vi "HTTP-Read Response.vi"(8 "error in (no error)":errorcluster, 11 "TCP Network Connection in":refnum<k5>) -> (0 "error out":errorcluster, 1 "Body":string, 2 "Header":string, 3 "TCP Network Connection out":refnum<k5>)   [LabVIEW 2020]
uses:
  <vilib>/regexp/Match Regular Expression.xnode
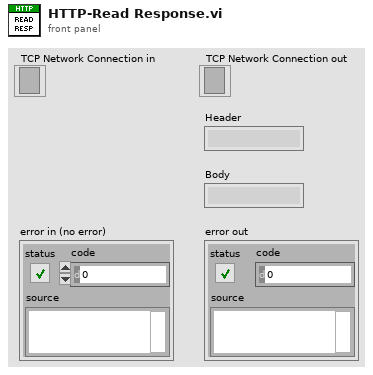
[diagram p1: front panel]
types:
  T1 = enum16{"Standard", "Buffered", "CRLF", "Immediate"}
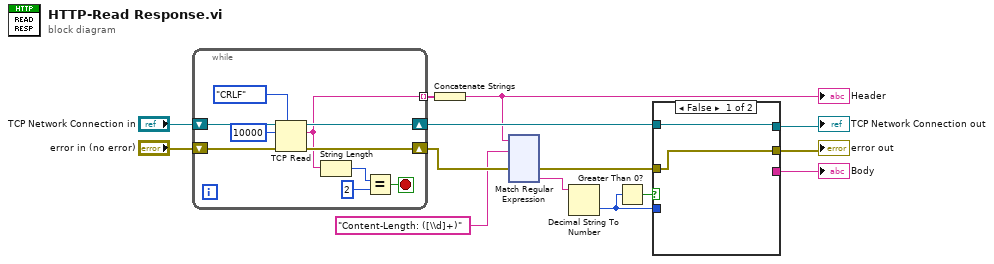
[diagram p0: block diagram]
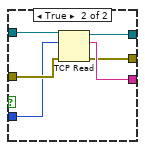
[diagram p2: hidden frame]
diagram:
  n1 = while {
    tunnel: [w18] -> w10 mode=indexing
    shift-right: [w21] -> w7
    shift-left: "error in (no error)" -> [w24]
    shift-right: [w20] -> w11
    shift-left: "TCP Network Connection in" -> [w23]
    stop <- w17 stop-if-true
    n2 = TCP Read(connection ID=w23, bytes to read=10000, error in (no error)=w24, 7:T1."CRLF" ("mode (standard)")) -> (connection ID out=w20:refnum<k5>, data out=w18:string, error out=w21:errorcluster)  [unwired: 1 in]
    n3 = String Length(string=w18) -> (length=w16:i32)
    n4 = Equal?(x=w16, y=2) -> (x = y?=w17:bool)
  }
  n5 = Concatenate Strings(w10) -> (w5:string)
  "Header" <- w5
  n6 = xnode "Match Regular Expression"("input string"=w5, "regular expression"="Content-Length: ([\\d]+)", "error in"=w7) -> ("error out"=w6:errorcluster, "submatch 1"=w3:string)  [unwired: 3 in, 4 out]
  n7 = Decimal String To Number(string=w3) -> (number=w1:i32)  [unwired: 2 in, 1 out]
  n8 = Greater Than 0?(x=w1) -> (x > 0?=w2:bool)
  n9 = case shown="False" w2 {
    tunnel: [_ w32] -> w14
    tunnel: [w25 w31] -> w13
    tunnel: [w26 w30] -> w12
    tunnel: w11 -> [w26 w29]
    tunnel: w6 -> [w25 w28]
    tunnel: w1 -> [_ w27]
    frame False {
    }
    frame True {
      n10 = TCP Read(connection ID=w29, bytes to read=w27, error in (no error)=w28) -> (connection ID out=w30:refnum<k5>, data out=w32:string, error out=w31:errorcluster)  [unwired: 2 in]
    }
  }
  "Body" <- w14
  "error out" <- w13
  "TCP Network Connection out" <- w12
